vi "Exercise 3-9.vi"(9 "Max Temp":dbl, 10 "Min Temp":dbl, 11 "Current Temp":dbl) -> (1 "Warning?":bool, 2 "Warning Text":string)   [LabVIEW 2014]
doc: "This VI is an exercise in the LabVIEW Core I course. During this exercise, you modify the code to use a Formula Node and/or a Case structure."
panel:
  in  "Max Wind Speed":dbl
  in  "Current Wind Speed":dbl
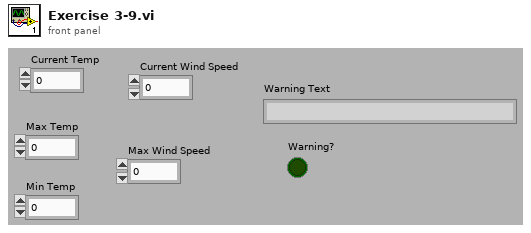
[diagram p1: front panel]
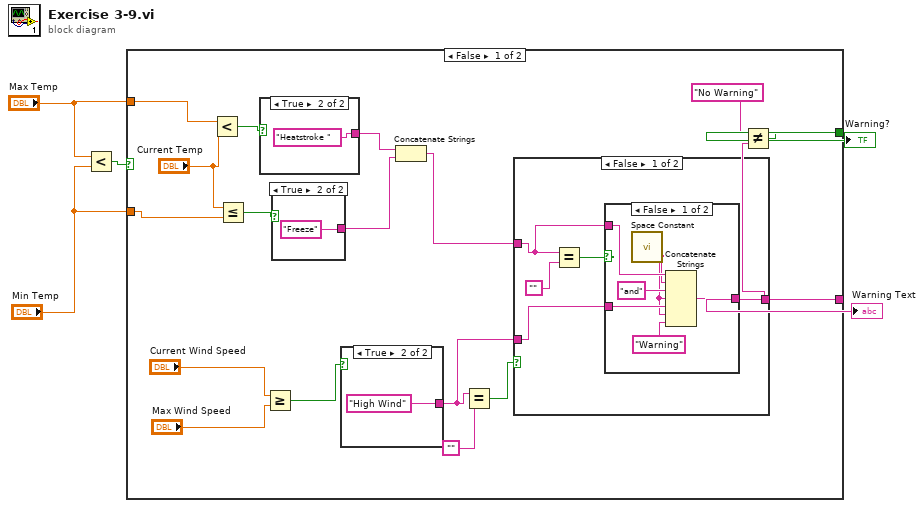
[diagram p0: block diagram]
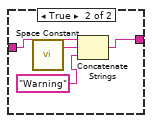
[diagram p2: hidden frame]
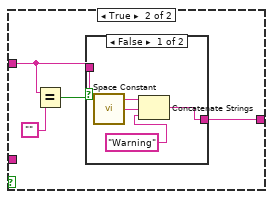
[diagram p3: hidden frame]
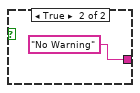
[diagram p4: hidden frame]
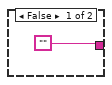
[diagram p5: hidden frame]
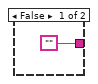
[diagram p6: hidden frame]
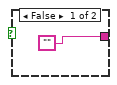
[diagram p7: hidden frame]
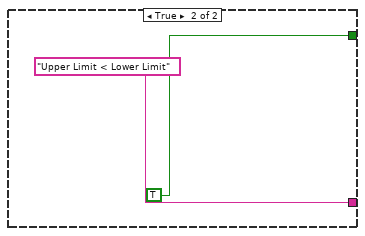
[diagram p8: hidden frame]
diagram:
  n1 = Less?(x="Max Temp", y="Min Temp") -> (x < y?=w3:bool)
  n2 = case shown="False" w3 {
    tunnel: [w12 "Upper Limit < Lower Limit" ("f")] -> w5
    tunnel: [w14 TRUE] -> w4
    tunnel: "Min Temp" -> [w21 _]
    tunnel: "Max Temp" -> [w22 _]
    frame False {
      n3 = Less?(x=w22, y="Current Temp") -> (x < y?=w18:bool)
      n4 = Less Or Equal?(x="Current Temp", y=w21) -> (x <= y?=w19:bool)
      n5 = case shown="True" w18 {
        tunnel: ["" "Heatstroke "] -> w11
        frame False {
        }
        frame True {
        }
      }
      n6 = Greater Or Equal?(x="Current Wind Speed", y="Max Wind Speed") -> (x >= y?=w17:bool)
      n7 = case shown="True" w19 {
        tunnel: ["" "Freeze"] -> w10
        frame False {
        }
        frame True {
        }
      }
      n8 = case shown="True" w17 {
        tunnel: ["" "High Wind"] -> w6
        frame False {
        }
        frame True {
        }
      }
      n9 = Concatenate Strings(w11, w10) -> (w9:string)
      n10 = Equal?(x=w6, y="") -> (x = y?=w8:bool)
      n11 = case shown="False" w8 {
        tunnel: [w24 w38] -> w12
        tunnel: w9 -> [w25 w40]
        tunnel: w6 -> [w23 _]
        frame False {
          n12 = Equal?(x=w25, y="") -> (x = y?=w26:bool)
          n13 = case shown="False" w26 {
            tunnel: w25 -> [w32 _]
            tunnel: [w33 w37] -> w24
            tunnel: w23 -> [w30 w36]
            frame False {
              n14 = call <vilib>:"Space Constant.vi"() -> ("String"=w29:string)
              n15 = Concatenate Strings(w32, w29, "and", w29, w30, w29, "Warning") -> (w33:string)
            }
            frame True {
              n16 = call <vilib>:"Space Constant.vi"() -> ("String"=w35:string)
              n17 = Concatenate Strings(w36, w35, "Warning") -> (w37:string)
            }
          }
        }
        frame True {
          n18 = Equal?(x=w40, y="") -> (x = y?=w41:bool)
          n19 = case shown="False" w41 {
            tunnel: w40 -> [w44 _]
            tunnel: [w42 "No Warning"] -> w38
            frame False {
              n20 = call <vilib>:"Space Constant.vi"() -> ("String"=w45:string)
              n21 = Concatenate Strings(w44, w45, "Warning") -> (w42:string)
            }
            frame True {
            }
          }
        }
      }
      n22 = Not Equal?(x="No Warning", y=w12) -> (x != y?=w14:bool)
    }
    frame True {
    }
  }
  "Warning Text" <- w5
  "Warning?" <- w4
